vi "GetAutoMode.vi"   [LabVIEW 2013]
uses:
  Robot Global Data.vi
types:
  T1 = typedef "Autonomous Data.ctl" = cluster{"Auto Mode":enum16{"Do Nothing", "Drive Forward", "Wait For Hot", "Turn L To Hot", "Turn R To Hot", "Turn To Hot From Center", "Two Ball From Center", "Two Ball", ""}, "Delay (s)":dbl}
  T2 = enum16{"Do Nothing", "Drive Forward", "Wait For Hot", "Turn L To Hot", "Turn R To Hot", "Turn To Hot From Center", "Two Ball From Center", "Two Ball", ""}
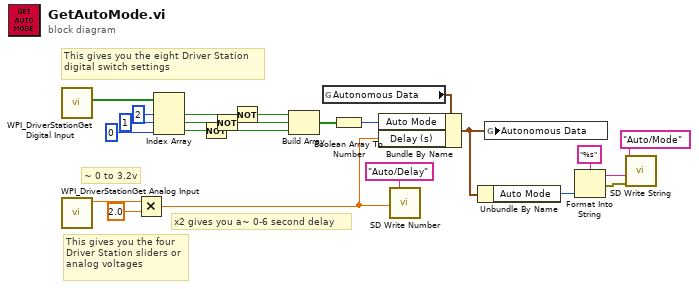
[diagram p0: block diagram]
diagram:
  # "~ 0 to 3.2v"
  # "x2 gives you a~ 0-6 second delay"
  # "This gives you the eight Driver Station\ndigital switch settings"
  # "This gives you the four\nDriver Station sliders or\nanalog voltages"
  n1 = call <vilib>:"WPI_DriverStationGet Digital Input.vi"() -> ("Driver Station Digital Input (1-8)"=w23:bool[])  [unwired: 11 out]
  n2 = call <vilib>:"WPI_DriverStationGet Analog Input.vi"() -> ("Analog 1 (V)"=w16:dbl)  [unwired: 11 out]
  n3 = Multiply(x=w16, y=2.0) -> (x*y=w8:dbl)
  n4 = Index Array(array=w23, index #1=2 ("index"), index #2=1 ("index"), index #3=0 ("index")) -> (element #1=w11:bool, element #2=w10:bool, element #3=w9:bool)
  n5 = Not(x=w9) -> (.not. x?=w12:bool)
  n6 = Not(x=w10) -> (.not. x?=w13:bool)
  n7 = Not(x=w11) -> (.not. x?=w14:bool)
  n8 = Build Array(w14, w13, w12) -> (w18:bool[])
  n9 = global read "Robot Global Data.vi" "Autonomous Data"() -> (w19:T1)
  n10 = Boolean Array To Number(Boolean array=w18) -> (number=w17:u32)
  n11 = Bundle By Name(cluster=w19, "Auto Mode"=w17, "Delay (s)"=w8) -> (w7:T1)
  n12 = call <vilib>:"SD Write Number.vi"("Numeric"=w8, "Name"="Auto/Delay") -> ()  [unwired: 8 in, 2 out]
  n13 = Unbundle By Name(w7) -> ("Auto Mode"=w5:T2)
  n14 = global write "Robot Global Data.vi" "Autonomous Data"(w7) -> ()
  n15 = Format Into String(format string="%s", w5) -> (resulting string=w2:string, error out=w3:errorcluster)  [unwired: 2 in]
  n16 = call <vilib>:"SD Write String.vi"("error in"=w3, "String"=w2, "Name"="Auto/Mode") -> ()  [unwired: 7 in, 2 out]
